vi "Main.vi"(10 "Mensajes Subpanel":refnum<vi>, 11 "Module Admin":refnum<class "Delacor_lib_QMH_Module Admin.lvclass">) -> ()   [LabVIEW 2020, in "Mensajes.lvlib"]
doc: "This template is based off of the Queued Message Handler design pattern and the Queued Message Handler project template that ships with LabVIEW.\n\nThe main difference is that the queue is private to this module and communication between modules is performed via Broadcast and Request events.\n\nRequest events are wrapped in public API methods and are handled in the Event Handling Loop (EHL) of this VI. Any module can register for Broadcast events sent by this module. The EHL generates messages based on user interface actions.\n\nThe Message Handling Loop (MHL) processes messages generated by the EHL, or by other messages. The messages are string values, so new messages can be added easily to the Message Cases case structure in the MHL. Each message cluster can also provide an optional value for Message Data, which is a variant that can be converted to whatever message-specific data is required.\n_____\nBased on Delacor QMH Project Template 5.0.0.82."
uses:
  Mensajes.lvlib
  <vilib>/Delacor/Delacor QMH/Libraries/Module Admin_class/Delacor_lib_QMH_Module Admin.lvclass
  Module Data--cluster.ctl
  Stop Argument--cluster.ctl
  <vilib>/Delacor/Delacor QMH/Libraries/Message Queue_class/Delacor_lib_QMH_Message Queue.lvclass/Delacor_lib_QMH_Message Queue.ctl
  <vilib>/Delacor/Delacor QMH/Libraries/Module Admin_class/Delacor_lib_QMH_Module Admin.lvclass/Delacor_lib_QMH_Module Admin.ctl
  Publicar mensaje Argument--cluster.ctl
  <vilib>/Utility/miscctls.llb/LVPointTypeDef.ctl
  <vilib>/Delacor/Delacor QMH/Libraries/Message Queue_class/Delacor_lib_QMH_Enqueue Message (Single).vi
  <vilib>/Delacor/Delacor QMH/Libraries/Module Admin_class/Delacor_lib_QMH_Get External Launch.vi
  <vilib>/Utility/error.llb/Error Cluster From Error Code.vi
  <vilib>/ErrorRing/Error Ring.xnode
  <vilib>/Delacor/Delacor QMH/Libraries/Message Queue_class/Delacor_lib_QMH_Message Queue.lvclass
panel:
  out "error out":errorcluster
  out "Status":string
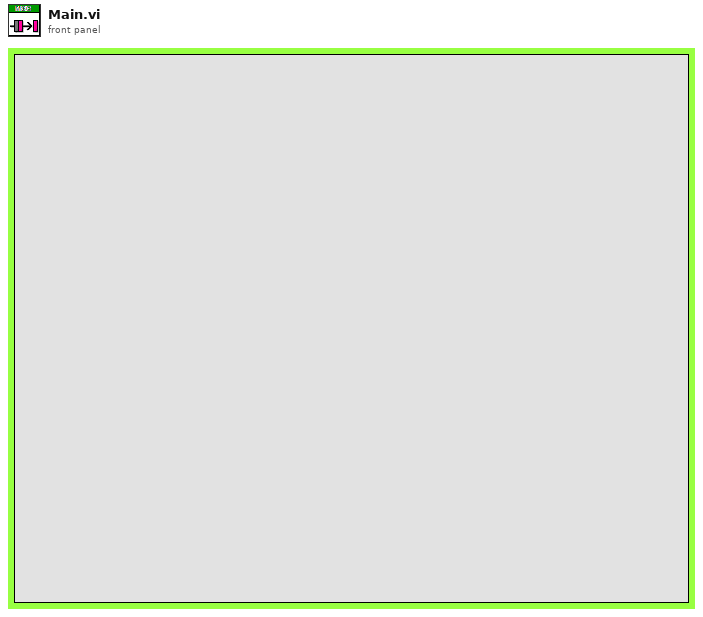
[diagram p1: front panel]
types:
  T1 = typedef "Mensajes.lvlib/Request Events--cluster.ctl" = cluster{"Stop Module":refnum<user-event>, "Show Panel":refnum<user-event>, "Hide Panel":refnum<user-event>, "Get Module Execution Status":refnum<user-event>, "Show Diagram":refnum<user-event>, "Publicar mensaje":refnum<user-event>}
  T2 = typedef "Mensajes.lvlib/Module Data--cluster.ctl" = cluster{"Status":string}
  T3 = enum32{"invalid lock state", "Not Locked", "Locked (No Password)", "Password-protected"}
  T4 = typedef "Mensajes.lvlib/Stop Argument--cluster.ctl" = cluster{"Origin":string, "Exit via Stop Module Req?":bool, "Wait for Module to stop?":bool}
  T5 = typedef "Mensajes.lvlib/Publicar mensaje Argument--cluster.ctl" = cluster{"Mensaje":string}
  T6 = typedef "LVPointTypeDef.ctl" = cluster{"Horizontal":i16, "Vertical":i16}
  T7 = enum32{"Invalid", "Standard", "Closed", "Hidden", "Minimized", "Maximized"}
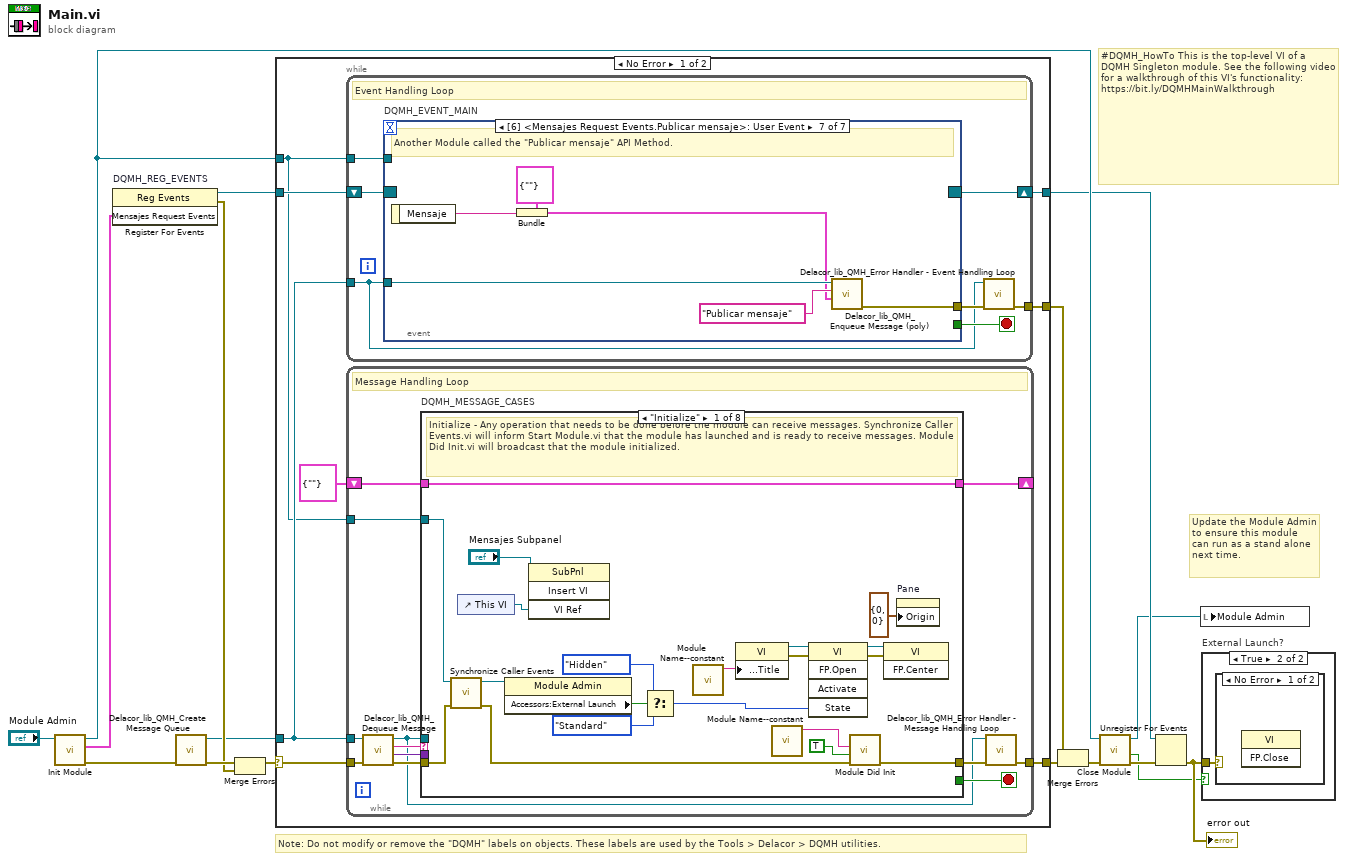
[diagram p0: block diagram]
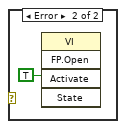
[diagram p3: hidden frame]
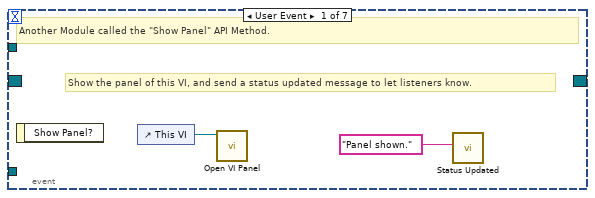
[diagram p4: hidden frame]
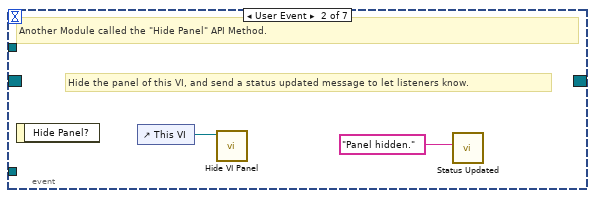
[diagram p5: hidden frame]
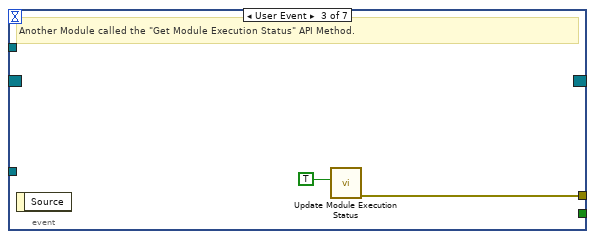
[diagram p6: hidden frame]
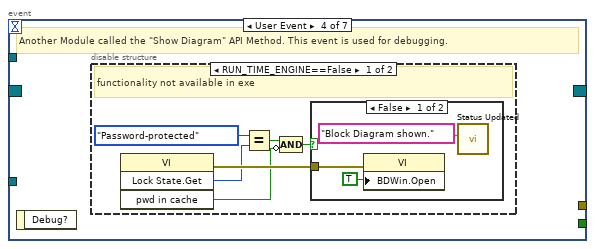
[diagram p7: hidden frame]
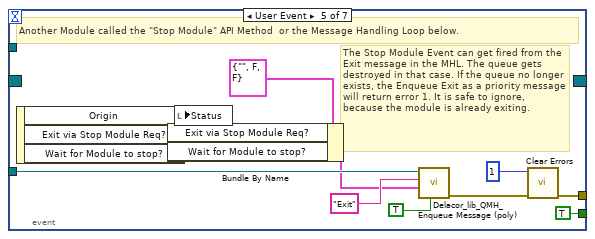
[diagram p10: hidden frame]
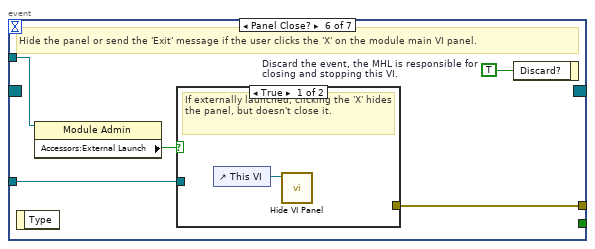
[diagram p11: hidden frame]
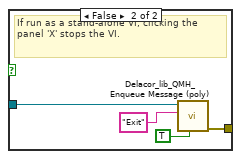
[diagram p12: hidden frame]
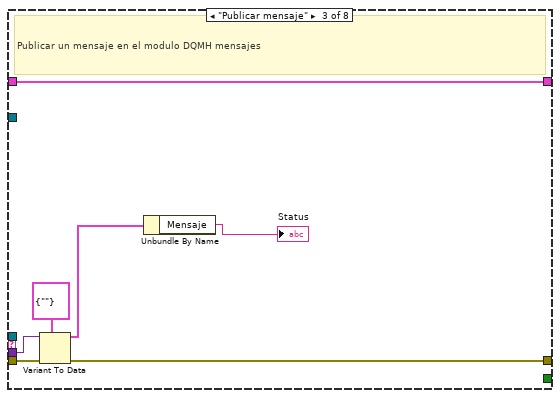
[diagram p14: hidden frame]
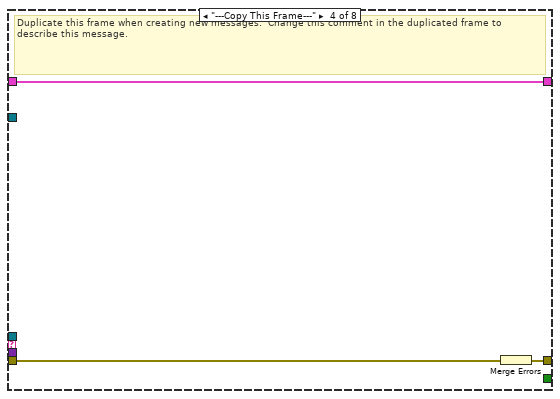
[diagram p15: hidden frame]
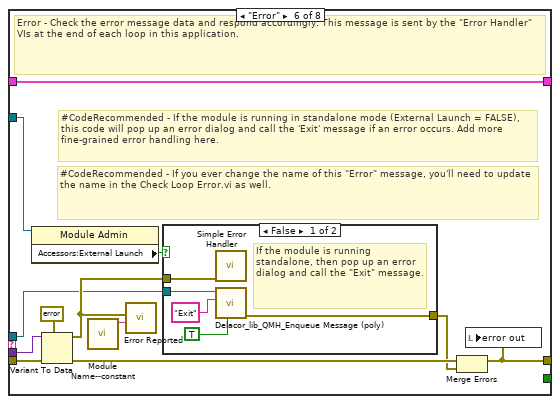
[diagram p17: hidden frame]
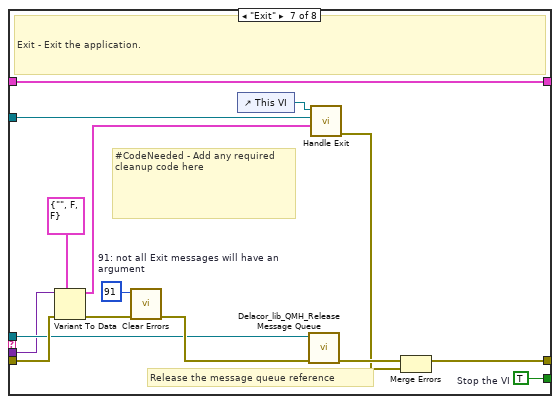
[diagram p19: hidden frame]
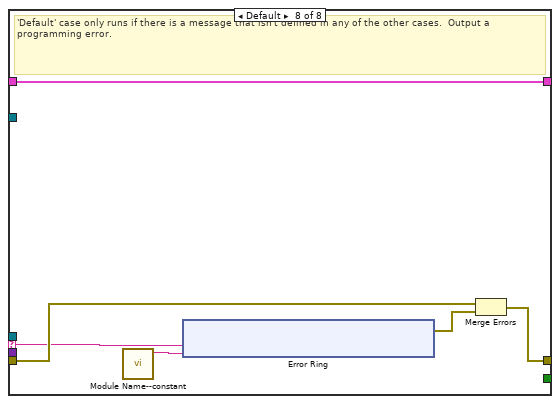
[diagram p20: hidden frame]
diagram:
  # "#DQMH_HowTo This is the top-level VI of a DQMH Singleton module. See the following video for a walkthrough of this VI's functionality: https://bit.ly/DQMHMainWalkthrough"
  # "Note: Do not modify or remove the \"DQMH\" labels on objects. These labels are used by the Tools > Delacor > DQMH utilities."
  # "Update the Module Admin to ensure this module can run as a stand alone next time."
  n1 = call "Init Module.vi"("Singleton Module Admin in"="Module Admin") -> ("error out"=w16:errorcluster, "Mensajes Request Events"=w5:T1, "Singleton Module Admin out"=w8:refnum<class "Delacor_lib_QMH_Module Admin.lvclass">)  [unwired: 8 in]
  n2 = register-events "DQMH_REG_EVENTS"(w5) -> (reference out=w6:refnum<event-registration>, error out=w9:errorcluster)  [unwired: 2 in]
  n3 = call <vilib>:"Delacor_lib_QMH_Create Message Queue.vi"("error in (no error)"=w16) -> ("error out"=w11:errorcluster, "Message Queue"=w4:refnum<class "Delacor_lib_QMH_Message Queue.lvclass">)  [unwired: 9 in]
  n4 = Merge Errors(w11, w9) -> (w10:errorcluster)
  n5 = case shown="No Error" w10 {
    selector: w10 -> [w23 w170]
    tunnel: [w25 w169] -> w17
    tunnel: [w22 w175] -> w7
    tunnel: w6 -> [w20 w175]
    tunnel: w4 -> [w19 w168]
    tunnel: [w24 _] -> w14
    tunnel: w8 -> [w18 w171]
    frame No Error {
      n6 = while {
        tunnel: w19 -> [w26]
        shift-right: [w29] -> w22
        shift-left: w20 -> [w30]
        tunnel: [w31] -> w24
        tunnel: w18 -> [w27]
        stop <- w28 stop-if-true
        # "Event Handling Loop"
        n7 = event "DQMH_EVENT_MAIN" shown="[6] <Mensajes Request Events.Publicar mensaje>: User Event" {
          selector: w30 -> [_ _ _ _ _ _ _]
          dyn-events: [_ _ _ _ _ _ _] -> w29
          timeout: _ -> [_ _ _ _ _ _ _]
          tunnel: [_ _ _ _ TRUE ("Discard?") _ _] -> w28
          tunnel: w26 -> [_ _ _ _ w55 w62 w75]
          tunnel: [_ _ w38 _ w58 w64 w70] -> w32
          tunnel: w27 -> [_ _ _ _ _ w61 _]
          event User Event {
            # "Show the panel of this VI, and send a status updated message to let listeners know."
            # "Another Module called the \"Show Panel\" API Method."
            n8 = event-data() -> ()  [unwired: 1 in, 1 out]
            n9 = control-ref of="This VI"() -> (w34:refnum<vi>)
            n10 = call "Open VI Panel.vi"("VI"=w34) -> ()  [unwired: 10 in, 1 out]
            n11 = call "Status Updated.vi"("Status"="Panel shown." ("format string")) -> ()  [unwired: 10 in, 1 out]
          }
          event User Event {
            # "Hide the panel of this VI, and send a status updated message to let listeners know."
            # "Another Module called the \"Hide Panel\" API Method."
            n12 = event-data() -> ()  [unwired: 1 in, 1 out]
            n13 = control-ref of="This VI"() -> (w36:refnum<vi>)
            n14 = call "Hide VI Panel.vi"("VI"=w36) -> ()  [unwired: 10 in, 1 out]
            n15 = call "Status Updated.vi"("Status"="Panel hidden." ("format string")) -> ()  [unwired: 10 in, 1 out]
          }
          event User Event {
            # "Another Module called the \"Get Module Execution Status\" API Method."
            n16 = event-data() -> ()  [unwired: 1 in, 1 out]
            n17 = call "Update Module Execution Status.vi"("Running?"=TRUE) -> ("error out"=w38:errorcluster)  [unwired: 10 in]
          }
          event User Event {
            # "Another Module called the \"Show Diagram\" API Method. This event is used for debugging."
            n18 = event-data() -> ()  [unwired: 1 in, 1 out]
            n19 = disable-structure shown="RUN_TIME_ENGINE==False" {
              frame condition #0 (active) {
                # "functionality not available in exe"
                n20 = invoke class="VI" method="Lock State.Get"() -> (error out=w44:errorcluster, "Get Lock State"=w43:T3, "pwd in cache"=w40:bool)  [unwired: 4 in, 1 out]
                n21 = Equal?(x=T3."Password-protected", y=w43) -> (x = y?=w41:bool)
                n22 = Compound Arithmetic op=AND(w41, invert w40) -> (w39:bool)
                n23 = case shown="False" w39 {
                  tunnel: w44 -> [w47 _]
                  frame False {
                    n24 = property class="VI"(error in=w47, "BDWin.Open"=TRUE ("Block Diagram Window:Open")) -> ()  [unwired: 1 in, 2 out]
                    n25 = call "Status Updated.vi"("Status"="Block Diagram shown." ("format string")) -> ()  [unwired: 10 in, 1 out]
                  }
                  frame True {
                    # "Password-protected VI, and the password is not in the cache. Do not show the diagram."
                  }
                }
              }
              frame condition #1 {
              }
            }
          }
          event User Event {
            # "The Stop Module Event can get fired from the Exit message in the MHL. The queue gets destroyed in that case. If the queue no longer exists, the Enqueue Exit as a priority message will return error 1. It is safe to ignore, because the module is already exiting."
            # "Another Module called the \"Stop Module\" API Method  or the Message Handling Loop below."
            n26 = event-data() -> ("Origin"=w54:string, "Exit via Stop Module Req?"=w50:bool, "Wait for Module to stop?"=w49:bool)  [unwired: 1 in]
            n27 = Bundle By Name(cluster=T4 {"Origin"="", "Exit via Stop Module Req?"=FALSE, "Wait for Module to stop?"=FALSE} ("Stop Argument"), "Exit via Stop Module Req?"=w50, "Wait for Module to stop?"=w49) -> (w48:T4)
            n28 = local write "Status"(w54) -> ()
            n29 = call-poly <vilib>:"Delacor_lib_QMH_Enqueue Message (poly).vi"("Priority Message? (F)"=TRUE, "Message Data"=w48, "Message"="Exit", "Message Queue in"=w55) -> ("error out"=w59:errorcluster)  [unwired: 6 in, 1 out]
            n30 = call <vilib>:"Clear Errors.vi"("error in (no error)"=w59, "specific error code to clear (0: all)"=1) -> ("error out"=w58:errorcluster)  [unwired: 4 in, 1 out]
          }
          event Panel Close? {
            w63 = TRUE  # Discard the event, the MHL is responsible for closing and stopping this VI.
            # "Hide the panel or send the 'Exit' message if the user clicks the 'X' on the module main VI panel."
            n31 = event-data() -> ()  [unwired: 1 in, 1 out]
            n32 = property class="Module Admin"(reference=w61) -> ("Accessors:External Launch"=w60:bool)  [unwired: 1 in, 2 out]
            n33 = case shown="True" w60 {
              tunnel: w62 -> [_ w68]
              tunnel: [_ w69] -> w64
              frame True {
                # "If externally launched, clicking the 'X' hides the panel, but doesn't close it."
                n34 = control-ref of="This VI"() -> (w65:refnum<vi>)
                n35 = call "Hide VI Panel.vi"("VI"=w65) -> ()  [unwired: 10 in, 1 out]
              }
              frame False {
                # "If run as a stand-alone VI, clicking the panel 'X' stops the VI."
                n36 = call-poly <vilib>:"Delacor_lib_QMH_Enqueue Message (poly).vi"("Priority Message? (F)"=TRUE, "Message"="Exit", "Message Queue in"=w68) -> ("error out"=w69:errorcluster)  [unwired: 7 in, 1 out]
              }
            }
            n37 = event-data("Discard?"=w63) -> ()  [unwired: 1 in, 1 out]
          }
          event User Event {
            # "Another Module called the \"Publicar mensaje\" API Method."
            n38 = event-data() -> ("Mensaje"=w71:string)  [unwired: 1 in]
            n39 = Bundle(cluster=T5 {"Mensaje"=""} ("Publicar mensaje Argument"), "Mensaje"=w71) -> (w72:T5)
            n40 = call-poly <vilib>:"Delacor_lib_QMH_Enqueue Message (poly).vi"("Message Data"=w72, "Message"="Publicar mensaje", "Message Queue in"=w75) -> ("error out"=w70:errorcluster)  [unwired: 7 in, 1 out]
          }
        }
        n41 = call-dynamic "Delacor_lib_QMH_Error Handler - Event Handling Loop.vi"("error in (no error)"=w32, "Message Queue in"=w26) -> ("dup error in"=w31:errorcluster)  [unwired: 8 in, 1 out]
      }
      n42 = while {
        tunnel: w19 -> [w78]
        shift-right: [w82] -> _
        shift-left: T2 {"Status"=""} ("Data Cluster") -> [w83]
        tunnel: w23 -> [w86]
        tunnel: [w84] -> w25
        tunnel: w18 -> [w76]
        stop <- w81 stop-if-true
        # "Message Handling Loop"
        n43 = call-dynamic "Delacor_lib_QMH_Dequeue Message.vi"("error in (no error)"=w86, "Message Queue in"=w78) -> ("error out"=w85:errorcluster, "Message Data"=w79:variant, "Message"=w80:string, "Message Queue out"=w77:refnum<class "Delacor_lib_QMH_Message Queue.lvclass">)  [unwired: 6 in]
        n44 = case "DQMH_MESSAGE_CASES" shown="\"Initialize\"" w80 {
          selector: w80 -> [_ _ _ _ _ _ _ w155]
          tunnel: w77 -> [_ _ _ _ _ w125 w147 _]
          tunnel: w85 -> [w105 w109 w116 w119 w121 w132 w153 w157]
          tunnel: [w103 w109 w114 w118 w121 w128 w150 w158] -> w87
          tunnel: w83 -> [w94 w108 w115 w117 w120 w127 w146 w156]
          tunnel: [w94 w108 w115 w117 w120 w127 w146 w156] -> w82
          tunnel: [_ _ _ _ _ _ w145 _] -> w81
          tunnel: w79 -> [_ _ w113 _ _ w126 w144 _]
          tunnel: w76 -> [w95 _ _ _ _ w124 w139 _]
          frame "Initialize" {
            # "Initialize - Any operation that needs to be done before the module can receive messages. Synchronize Caller Events.vi will inform Start Module.vi that the module has launched and is ready to receive messages. Module Did Init.vi will broadcast that the module initialized."
            n45 = call "Synchronize Caller Events.vi"("error in (no error)"=w105, "Singleton Module Admin in"=w95) -> ("error out"=w104:errorcluster, "Singleton Module Admin out"=w91:refnum<class "Delacor_lib_QMH_Module Admin.lvclass">)  [unwired: 8 in]
            n46 = control-ref of="This VI"() -> (w88:refnum<vi>)
            n47 = property class="Module Admin"(reference=w91) -> ("Accessors:External Launch"=w99:bool)  [unwired: 1 in, 2 out]
            n48 = invoke class="SubPnl" method="Insert VI"(reference="Mensajes Subpanel", "VI Ref"=w88) -> ()  [unwired: 2 in, 4 out]
            n49 = Select(t=T7."Hidden" ("State"), s=w99, f=T7."Standard" ("State")) -> (s? t:f=w96:T7)
            n50 = call "Module Name--constant.vi"() -> ("Module Name"=w102:string)  [unwired: 11 in]
            n51 = property class="VI"("Front Panel.Title"=w102) -> (reference out=w101:refnum<vi>, error out=w107:errorcluster)  [unwired: 2 in]
            n52 = call "Module Name--constant.vi"() -> ("Module Name"=w92:string)  [unwired: 11 in]
            n53 = invoke class="VI" method="FP.Open"(reference=w101, error in=w107, "State"=w96) -> (reference out=w100:refnum<vi>, error out=w106:errorcluster)  [unwired: 2 in, 3 out]
            n54 = call "Module Did Init.vi"("error in (no error)"=w104, "Initialized?"=TRUE, "Origin"=w92) -> ("error out"=w103:errorcluster)  [unwired: 8 in]
            n55 = invoke class="VI" method="FP.Center"(reference=w100, error in=w106) -> ()  [unwired: 1 in, 3 out]
            n56 = property on="Pane" class="Pane"("Origin"=T6 {"Horizontal"=0, "Vertical"=0}) -> ()  [unwired: 2 in, 2 out]
          }
          frame "--- Module Specific ---" {
            # "Separator -- The following cases handle messages specific to this Module."
          }
          frame "Publicar mensaje" {
            # "Publicar un mensaje en el modulo DQMH mensajes"
            n57 = Variant To Data(error in=w116, type=T5 {"Mensaje"=""} ("Publicar mensaje Argument"), Variant=w113) -> (data=w111:T5, error out=w114:errorcluster)
            n58 = Unbundle By Name(w111) -> ("Mensaje"=→"Status":string)
          }
          frame "---Copy This Frame---" {
            # "Duplicate this frame when creating new messages.  Change this comment in the duplicated frame to describe this message."
            n59 = Merge Errors(w119) -> (w118:errorcluster)
          }
          frame "--- Exit and Error Handling---" {
            # "Separator - The following cases handle errors and exit messages."
          }
          frame "Error" {
            # "#CodeRecommended - If you ever change the name of this \"Error\" message, you'll need to update the name in the Check Loop Error.vi as well."
            # "#CodeRecommended - If the module is running in standalone mode (External Launch = FALSE), this code will pop up an error dialog and call the 'Exit' message if an error occurs. Add more fine-grained error handling here."
            # "Error - Check the error message data and respond accordingly. This message is sent by the \"Error Handler\" VIs at the end of each loop in this application."
            n60 = property class="Module Admin"(reference=w124) -> ("Accessors:External Launch"=w123:bool)  [unwired: 1 in, 2 out]
            n61 = Variant To Data(error in=w132, type=errorcluster {"status"=FALSE, "code"=0, "source"=""} ("error constant"), Variant=w126) -> (data=w133:errorcluster, error out=w130:errorcluster)
            n62 = call "Module Name--constant.vi"() -> ("Module Name"=w122:string)  [unwired: 11 in]
            n63 = call "Error Reported.vi"("Additional Information"=w122, "Error"=w133) -> ()  [unwired: 9 in, 1 out]
            n64 = case shown="False" w123 {
              tunnel: [w138 _] -> w129
              tunnel: w125 -> [w136 _]
              tunnel: w133 -> [w137 _]
              frame False {
                # "If the module is running standalone, then pop up an error dialog and call the \"Exit\" message."
                n65 = call <vilib>:"Simple Error Handler.vi"("error in (no error)"=w137) -> ()  [unwired: 4 in, 5 out]
                n66 = call-poly <vilib>:"Delacor_lib_QMH_Enqueue Message (poly).vi"("Priority Message? (F)"=TRUE, "Message"="Exit", "Message Queue in"=w136) -> ("error out"=w138:errorcluster)  [unwired: 7 in, 1 out]
              }
              frame True {
                # "If the module was launched externally, calling the Error Reported broadcast VI is the only action performed by the \"Error\" message. The module's caller can then process the error appropriately."
              }
            }
            n67 = Merge Errors(w130, w129) -> (w128:errorcluster)
            n68 = local write "error out"(w128) -> ()
          }
          frame "Exit" {
            w143 = 91  # 91: not all Exit messages will have an argument
            w145 = TRUE  # Stop the VI
            # "Release the message queue reference"
            # "#CodeNeeded - Add any required cleanup code here"
            # "Exit - Exit the application."
            n69 = Variant To Data(error in=w153, type=T4 {"Origin"="", "Exit via Stop Module Req?"=FALSE, "Wait for Module to stop?"=FALSE} ("Stop Argument"), Variant=w144) -> (data=w141:T4, error out=w149:errorcluster)
            n70 = call <vilib>:"Clear Errors.vi"("error in (no error)"=w149, "specific error code to clear (0: all)"=w143) -> ("error out"=w152:errorcluster)  [unwired: 4 in, 1 out]
            n71 = control-ref of="This VI"() -> (w140:refnum<vi>)
            n72 = call-dynamic "Delacor_lib_QMH_Release Message Queue.vi"("error in (no error)"=w152, "Message Queue"=w147) -> ("error out"=w151:errorcluster)  [unwired: 9 in]
            n73 = call "Handle Exit.vi"("Stop Argument"=w141, "Admin in"=w139, "VI reference"=w140) -> ("error out"=w148:errorcluster)  [unwired: 7 in, 1 out]
            n74 = Merge Errors(w151, w148) -> (w150:errorcluster)
          }
          frame Default {
            # "'Default' case only runs if there is a message that isn't defined in any of the other cases.  Output a programming error."
            n75 = call "Module Name--constant.vi"() -> ("Module Name"=w154:string)  [unwired: 11 in]
            n76 = xnode "Error Ring"("parameter 0"=w155, "parameter 1"=w154) -> ("error out"=w159:errorcluster)
            n77 = Merge Errors(w157, w159) -> (w158:errorcluster)
          }
        }
        n78 = call-dynamic "Delacor_lib_QMH_Error Handler - Message Handling Loop.vi"("error in (no error)"=w87, "Message Queue in"=w77) -> ("dup error in"=w84:errorcluster)  [unwired: 8 in, 1 out]
      }
    }
    frame Error {
      # "Synchronize Caller Events.vi will inform Start Module.vi that the module has launched and will let the code calling Start Module.vi register for broadcasts and would permit the caller receive the broadcast that an error occurred at launch time."
      n79 = call-dynamic "Delacor_lib_QMH_Release Message Queue.vi"("error in (no error)"=w170, "Message Queue"=w168) -> ("error out"=w169:errorcluster)  [unwired: 9 in]
      n80 = call "Synchronize Caller Events.vi"("Singleton Module Admin in"=w171) -> ("error out"=w176:errorcluster)  [unwired: 9 in, 1 out]
      n81 = call "Module Name--constant.vi"() -> ("Module Name"=w174:string)  [unwired: 11 in]
      n82 = Format Into String(format string="An error occurred during initialization. %s is no longer running.", w174) -> (resulting string=w172:string)  [unwired: 2 in, 1 out]
      n83 = Merge Errors(w169, w176) -> (w177:errorcluster)
      n84 = call "Error Reported.vi"("Additional Information"=w172, "Error"=w177) -> ()  [unwired: 9 in, 1 out]
    }
  }
  n85 = Merge Errors(w14, w17) -> (w13:errorcluster)
  n86 = call "Close Module.vi"("error in (no error)"=w13, "Module Admin in"=w8) -> ("error out"=w15:errorcluster, "External Launch"=w1:bool, "Module Admin out"=w2:refnum<class "Delacor_lib_QMH_Module Admin.lvclass">)  [unwired: 7 in]
  n87 = Unregister For Events(event registration refnum=w7, error in=w15) -> (error out=w12:errorcluster)
  "error out" <- w12
  n88 = local write "Module Admin"(w2) -> ()
  n89 = case "External Launch?" shown="True" w1 {
    tunnel: w12 -> [_ w178]
    frame False {
    }
    frame True {
      n90 = case shown="No Error" w178 {
        frame No Error {
          n91 = invoke class="VI" method="FP.Close"() -> ()  [unwired: 3 in, 3 out]
        }
        frame Error {
          n92 = invoke class="VI" method="FP.Open"("Activate"=TRUE ("Activate?")) -> ()  [unwired: 4 in, 5 out]
        }
      }
    }
  }
